vi "Pop Up Before.vi"(10 "mode":T1) -> ()   [LabVIEW 2019, in "LSS.lvlib"]
doc: "Pop up dialog from the example done using property nodes.\n\n<b>Inputs:</b>\n<b>mode</b> - Used to select between different styles available for the pop up dialog."
uses:
  LSS.lvlib
  Themes.ctl
  Before UI References.ctl
  <vilib>/Utility/miscctls.llb/LVBoundsTypeDef.ctl
panel:
  in  "Button4":bool
  in  "Button3":bool
  in  "Button2":bool
  in  "Button1":bool
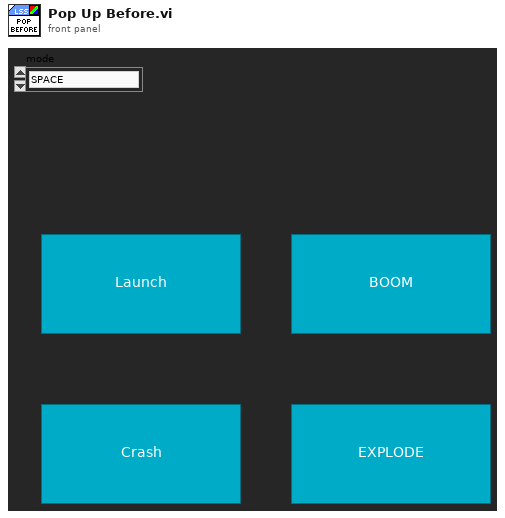
[diagram p1: front panel]
types:
  T1 = typedef "LSS.lvlib/Themes.ctl" = enum16{"SPACE", "ATK", "THEME1", "THEME2"}
  T2 = typedef "LVBoundsTypeDef.ctl" = cluster{"Width":u32, "Height":u32}
  T3 = typedef "LSS.lvlib/Before UI References.ctl" = cluster{"Panes":refnum<vi>[], "Splitter":refnum<vi>, "Mars Picture":refnum<vi>, "Buttons":refnum<vi>[], "Numerics":refnum<vi>[], "Graphs":refnum<vi>[], "Slides":refnum<vi>[], "This VI":refnum<vi>, "Vortex":refnum<vi>, "Map":refnum<vi>}
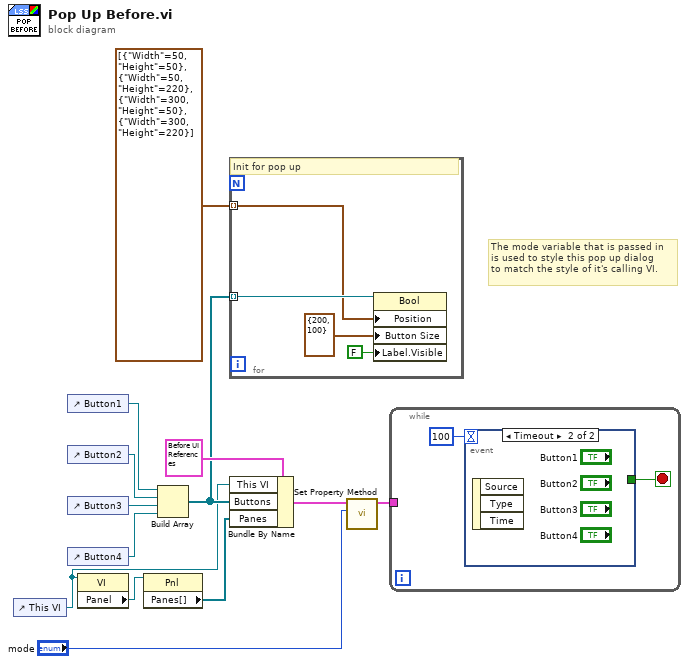
[diagram p0: block diagram]
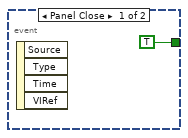
[diagram p2: hidden frame]
diagram:
  # "The mode variable that is passed in\nis used to style this pop up dialog\nto match the style of it's calling VI."
  n1 = control-ref of="This VI"() -> (w3:refnum<vi>)
  n2 = control-ref of="Button1"() -> (w7:refnum<vi>)
  n3 = control-ref of="Button2"() -> (w6:refnum<vi>)
  n4 = control-ref of="Button3"() -> (w5:refnum<vi>)
  n5 = control-ref of="Button4"() -> (w4:refnum<vi>)
  n6 = property class="VI"(reference=w3) -> ("Panel"=w2:refnum<vi>)  [unwired: 1 in, 2 out]
  n7 = property class="Pnl"(reference=w2) -> ("Panes[]"=w1:refnum<vi>[])  [unwired: 1 in, 2 out]
  n8 = Build Array(w7, w6, w5, w4) -> (w8:refnum<vi>[])
  n9 = for {
    tunnel: w8 -> [w17] mode=indexing
    tunnel: T2[] [{"Width"=50, "Height"=50}, {"Width"=50, "Height"=220}, {"Width"=300, "Height"=50}, {"Width"=300, "Height"=220}] ("Button Size") -> [w16] mode=indexing
    # "Init for pop up"
    n10 = property on="Property Node" class="Bool"(reference=w17, "Position"=w16, "Button Size"=T2 {"Width"=200, "Height"=100}, "Label.Visible"=FALSE) -> ()  [unwired: 1 in, 2 out]
  }
  n11 = Bundle By Name(cluster=T3 {"Panes"=[refnum, refnum], "Splitter"=refnum, "Mars Picture"=refnum, "Buttons"=[refnum, refnum, refnum, refnum, refnum, refnum], "Numerics"=[refnum, refnum, refnum, refnum], "Graphs"=[refnum, refnum, refnum], "Slides"=[refnum, refnum], "This VI"=refnum, "Vortex"=refnum, "Map"=refnum} ("Cluster"), "This VI"=w3, "Buttons"=w8, "Panes"=w1) -> (w12:T3)
  n12 = call "Set Property Method.vi"("Theme Choice"="mode", "Cluster"=w12) -> ("Cluster Out"=w10:T3)  [unwired: 9 in]
  n13 = while {
    tunnel: w10 -> [_]
    stop <- w18 stop-if-true
    n14 = event shown="[1] Timeout" {
      selector: _ -> [_ _]
      dyn-events: _ -> [_ _]
      timeout: 100 -> [_ _]
      tunnel: [TRUE _] -> w18
      event Panel Close {
        n15 = event-data() -> ()  [unwired: 1 in, 4 out]
      }
      event Timeout {
        n16 = event-data() -> ()  [unwired: 1 in, 3 out]
      }
    }
  }
